vi "Controller.vi"() -> ()   [LabVIEW 2025]
uses:
  Cluster.ctl
  Enum.ctl
  Conn_state.ctl
  <vilib>/Instr/_visa.llb/VISA Configure Serial Port (Instr).vi
  <vilib>/FPGAPlugInAG/myRIO-1900/niLvFpga_Open_myRIO-1900.vi
  <vilib>/rvi/interface/common/dynamic/niFpgaDynamicAddResources.vi
  <vilib>/Utility/error.llb/Error Cluster From Error Code.vi
  <vilib>/rvi/errors/niLvFpgaAdjustHostInterfaceError.vi
  <vilib>/FPGAPlugInAG/Dynamic/niLvFpga_Close_Dynamic.vi
  <vilib>/rvi/interface/nirviOpenFPGA/nirviOpenFPGA.xnode
  FPGA Bitfiles/project_FPGATarget_fpgamain_qld3yE8o4VA.lvbitx
  <vilib>/rvi/interface/nirviReadWriteControl/nirviReadWriteControl.xnode
  <vilib>/rvi/interface/nirviCloseFPGA/nirviCloseFPGA.xnode
  <resource>/objmgr/ni.dex.rc
  <vilib>/rvi/interface/Simulation/niFpgaSimulationCallBeginRW.vi
  NiFpgaLv.dll
panel:
  out "TEMPERATURA":dbl
  in  "Acq_delay_start":u16=500
  out "Is Connected":bool
  out "Stop":bool
  out "Acq_Data":i16[](graph)
  out "error out":errorcluster
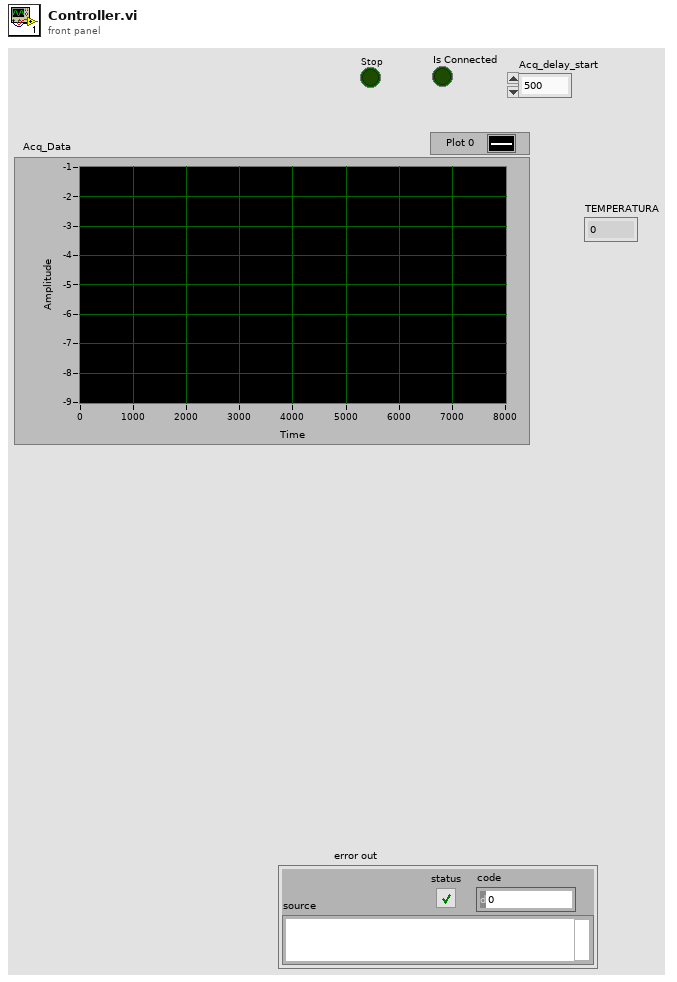
[diagram p1: front panel]
types:
  T1 = typedef "Conn_state.ctl" = enum16{"Disconected", "Reconecting", "Connected"}
  T2 = typedef "Cluster.ctl" = cluster{"Stop":bool, "Trigger":bool, "Select":T3, "Acq Delay":u16}
  T3 = typedef "Enum.ctl" = enum16{"Trigger", "Stop", "Acq_del"}
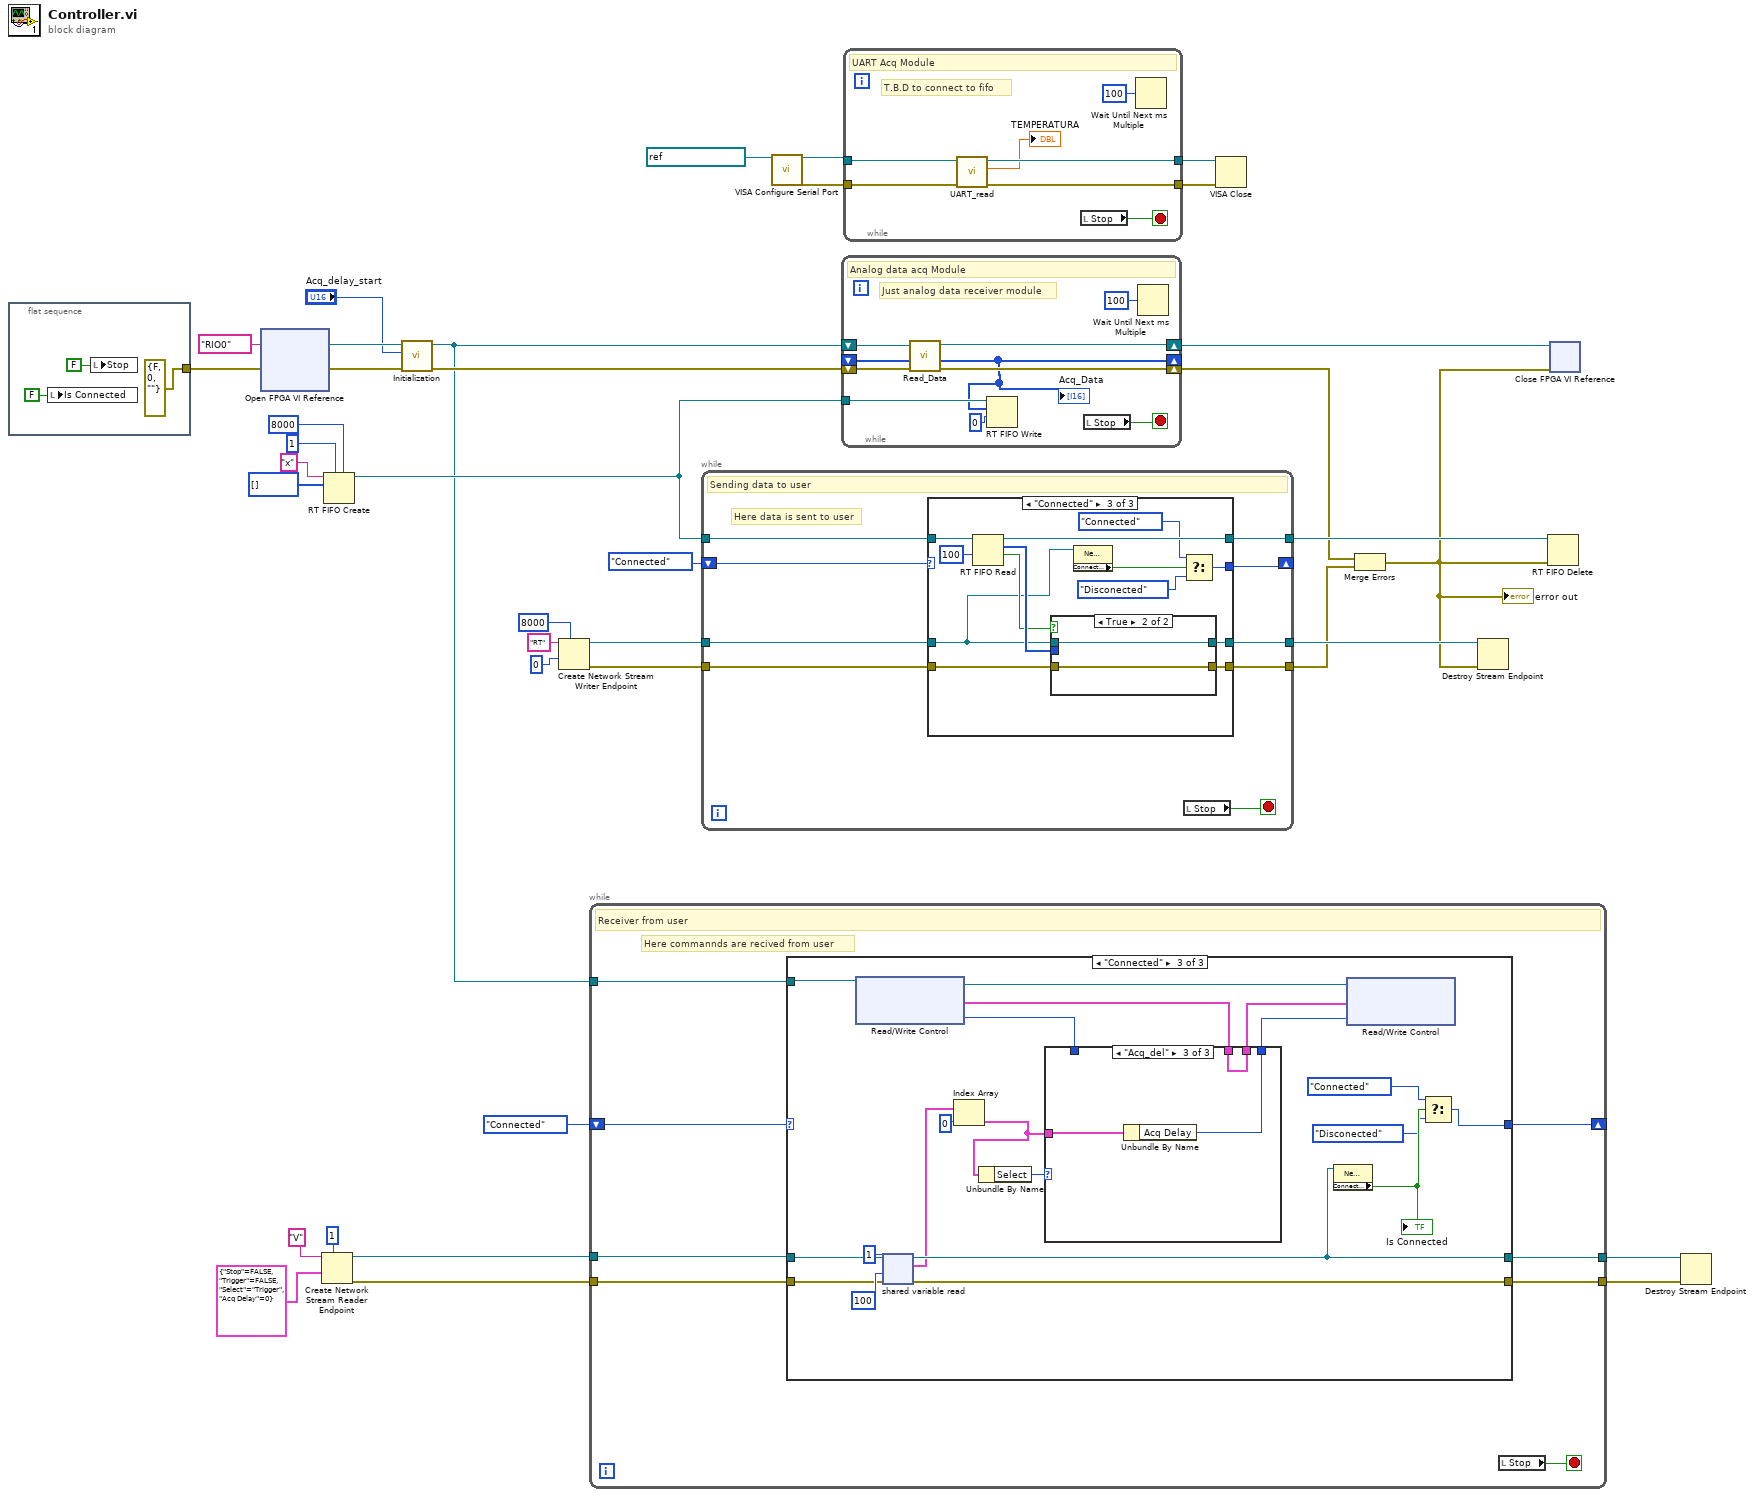
[diagram p0: block diagram]
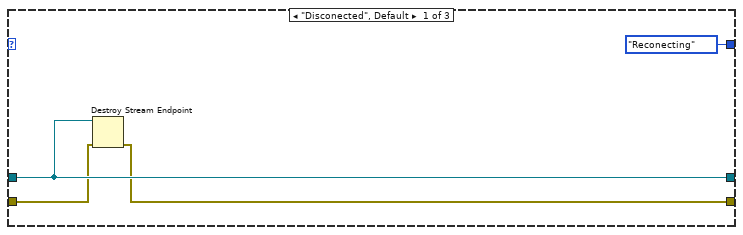
[diagram p2: hidden frame]
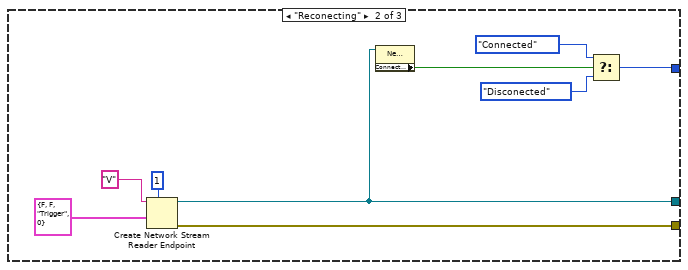
[diagram p3: hidden frame]
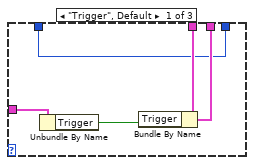
[diagram p4: hidden frame]
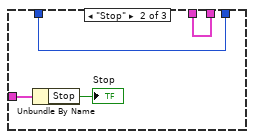
[diagram p5: hidden frame]
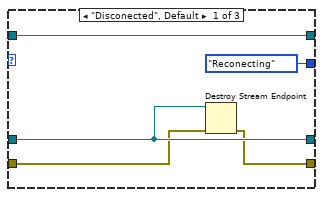
[diagram p6: hidden frame]
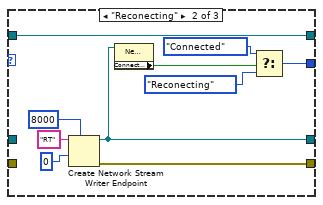
[diagram p7: hidden frame]
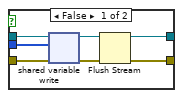
[diagram p8: hidden frame]
diagram:
  n1 = flat-sequence {
    tunnel: [errorcluster {"status"=FALSE, "code"=0, "source"=""} ("error in")] -> w26
    frame #0 {
      n2 = local write "Is Connected"(FALSE ("Is Connected")) -> ()
      n3 = local write "Stop"(FALSE ("Stop")) -> ()
    }
  }
  n4 = xnode "Open FPGA VI Reference"("error in"=w26, "resource name"=tag "RIO0") -> ("FPGA VI Reference Out"=w10:refnum<k20>, "error out"=w29:errorcluster)
  n5 = Create Network Stream Reader Endpoint(7:1 ("reader buffer size"), 9:T2 {"Stop"=FALSE, "Trigger"=FALSE, "Select"=enum."Trigger", "Acq Delay"=0} ("Variable"), 11:"V" ("reader name")) -> (0:w8:errorcluster, 3:w14:refnum<k21>)  [unwired: 4 in]
  n6 = RT FIFO Create(0:"x" ("name (unnamed)"), 1:i32[] [], 4:u32 1 ("size (10)"), 6:u32 8000 ("elements in array (1)")) -> (8:w32:refnum<k33>)  [unwired: 4 in, 2 out]
  n7 = call "Initialization.vi"("error in"=w29, "Acc_delay"="Acq_delay_start", "FPGA VI Reference In"=w10) -> ("error out"=w28:errorcluster, "FPGA VI Reference Out"=w6:refnum<k20>)  [unwired: 7 in]
  n8 = Create Network Stream Writer Endpoint(7:8000 ("writer buffer size"), 9:0, 11:"RT" ("writer name")) -> (0:w19:errorcluster, 3:w21:refnum<k21>)  [unwired: 4 in]
  n9 = while {
    tunnel: w6 -> [w48]
    tunnel: [w45] -> w17
    tunnel: w14 -> [w46]
    shift-right: [w43] -> _
    shift-left: Conn_state."Connected" ("Conn_state") -> [w44]
    tunnel: w8 -> [w42]
    tunnel: [w41] -> w7
    stop <- w47 stop-if-true
    # "Here commannds are recived from user"
    # "Receiver from user"
    n10 = case shown="\"Connected\"" w44 {
      tunnel: w48 -> [_ _ w81]
      tunnel: [w51 w54 w72] -> w45
      tunnel: w46 -> [w51 _ w70]
      tunnel: [Conn_state."Reconecting" ("Conn_state") w58 w66] -> w43
      tunnel: w42 -> [w50 _ w65]
      tunnel: [w49 w53 w64] -> w41
      frame "Disconected", Default {
        n11 = Destroy Stream Endpoint(8:w50, 11:w51) -> (0:w49:errorcluster)
      }
      frame "Reconecting" {
        n12 = Create Network Stream Reader Endpoint(7:1 ("reader buffer size"), 9:T2 {"Stop"=FALSE, "Trigger"=FALSE, "Select"=enum."Trigger", "Acq Delay"=0} ("Variable"), 11:"V" ("reader name")) -> (0:w53:errorcluster, 3:w54:refnum<k21>)  [unwired: 4 in]
        n13 = property class="Network Stream Endpoint"(reference=w54) -> ("Connected"=w59:bool)  [unwired: 1 in, 2 out]
        n14 = Select(t=Conn_state."Connected" ("Conn_state"), s=w59, f=Conn_state."Disconected" ("Conn_state")) -> (s? t:f=w58:T1)
      }
      frame "Connected" {
        n15 = xnode "Read/Write Control"("FPGA VI Reference In"=w81) -> ("FPGA VI Reference Out"=w78:refnum<k20>, "Var data"=w77:cluster{"Placeholder":i16, "Trigger":bool}, "Time Delay_Read"=w63:u16)  [unwired: 1 in, 1 out]
        n16 = shared-variable-read(w70, w65, 100 ("timeout ms (-1)"), 1 ("# elements")) -> (w72:refnum<k21>, w64:errorcluster, w71:T2[])  [unwired: 1 out]
        n17 = Index Array(array=w71, index=0) -> (element=w75:T2)
        n18 = Unbundle By Name(w75) -> ("Select"=w74:T3)
        n19 = case shown="\"Acq_del\"" w74 {
          tunnel: [w84 w88 w92] -> w73
          tunnel: w75 -> [w86 w90 w93]
          tunnel: w77 -> [w83 w88 w92]
          tunnel: w63 -> [w82 w87 _]
          tunnel: [w82 w87 w91] -> w62
          frame "Trigger", Default {
            n20 = Unbundle By Name(w86) -> ("Trigger"=w85:bool)
            n21 = Bundle By Name(cluster=w83, "Trigger"=w85) -> (w84:cluster{"Placeholder":i16, "Trigger":bool})
          }
          frame "Stop" {
            n22 = Unbundle By Name(w90) -> ("Stop"=→"Stop":bool)
          }
          frame "Acq_del" {
            n23 = Unbundle By Name(w93) -> ("Acq Delay"=w91:u16)
          }
        }
        n24 = property class="Network Stream Endpoint"(reference=w72) -> ("Connected"=w69:bool)  [unwired: 1 in, 2 out]
        "Is Connected" <- w69
        n25 = xnode "Read/Write Control"("FPGA VI Reference In"=w78, "Var data"=w73, "Time Delay_Read"=w62) -> ()  [unwired: 1 in, 2 out]
        n26 = Select(t=Conn_state."Connected" ("Conn_state"), s=w69, f=Conn_state."Disconected" ("Conn_state")) -> (s? t:f=w66:T1)
      }
    }
    n27 = local read "Stop"() -> (w47:bool)
  }
  n28 = while {
    tunnel: w32 -> [w102]
    tunnel: [w101] -> w33
    shift-right: [w98] -> _
    shift-left: Conn_state."Connected" ("Conn_state") -> [w99]
    tunnel: w21 -> [w97]
    tunnel: [w96] -> w20
    tunnel: w19 -> [w95]
    tunnel: [w94] -> w18
    stop <- w100 stop-if-true
    # "Here data is sent to user"
    # "Sending data to user"
    n29 = case shown="\"Connected\"" w99 {
      tunnel: w102 -> [w107 w116 w130]
      tunnel: w95 -> [w104 _ w129]
      tunnel: [w105 w108 w128] -> w96
      tunnel: [w107 w116 w127] -> w101
      tunnel: [w103 w109 w126] -> w94
      tunnel: w97 -> [w105 _ w122]
      tunnel: [Conn_state."Reconecting" ("Conn_state") w117 w118] -> w98
      frame "Disconected", Default {
        n30 = Destroy Stream Endpoint(8:w104, 11:w105) -> (0:w103:errorcluster)
      }
      frame "Reconecting" {
        n31 = Create Network Stream Writer Endpoint(7:8000 ("writer buffer size"), 9:0, 11:"RT" ("writer name")) -> (0:w109:errorcluster, 3:w108:refnum<k21>)  [unwired: 4 in]
        n32 = property class="Network Stream Endpoint"(reference=w108) -> ("Connected"=w115:bool)  [unwired: 1 in, 2 out]
        n33 = Select(t=Conn_state."Connected" ("Conn_state"), s=w115, f=Conn_state."Reconecting" ("Conn_state")) -> (s? t:f=w117:T1)
      }
      frame "Connected" {
        n34 = RT FIFO Read(0:w130, 2:100 ("timeout in ms (0)")) -> (8:w127:refnum<k33>, 9:w125:i32[], 10:w123:bool)  [unwired: 2 in, 2 out]
        n35 = case shown="True" w123 {
          tunnel: w125 -> [w137 _]
          tunnel: w129 -> [w134 w138]
          tunnel: w122 -> [w133 w139]
          tunnel: [w132 w139] -> w128
          tunnel: [w131 w138] -> w126
          frame False {
            n36 = shared-variable-write(w133, w134, w137) -> (w136:refnum<k21>, w135:errorcluster)  [unwired: 1 in, 1 out]
            n37 = Flush Stream(8:w135, 11:w136) -> (0:w131:errorcluster, 3:w132:refnum<k21>)  [unwired: 2 in, 1 out]
          }
          frame True {
          }
        }
        n38 = property class="Network Stream Endpoint"(reference=w122) -> ("Connected"=w121:bool)  [unwired: 1 in, 2 out]
        n39 = Select(t=Conn_state."Connected" ("Conn_state"), s=w121, f=Conn_state."Disconected" ("Conn_state")) -> (s? t:f=w118:T1)
      }
    }
    n40 = local read "Stop"() -> (w100:bool)
  }
  n41 = call-poly "VISA Configure Serial Port"("VISA resource name"=refnum<visa-resource-name> "ASRL1::INSTR") -> ("VISA resource name out"=w2:refnum<visa-resource-name>, "error out"=w1:errorcluster)  [unwired: 13 in]
  n42 = while {
    shift-right: [w140] -> w31
    shift-left: w6 -> [w141]
    shift-right: [w147] -> w30
    shift-left: w28 -> [w146]
    tunnel: w32 -> [w148]
    shift-right: [w143] -> _
    shift-left: _ -> [w145]
    stop <- w142 stop-if-true
    # "Just analog data receiver module"
    # "Analog data acq Module"
    n43 = call "Read_Data.vi"("error in"=w146, "Shift_Register_In"=w145, "FPGA VI Reference In"=w141) -> ("error out"=w147:errorcluster, "Shift_Register_Out"=w143:i16[], "FPGA VI Reference Out 2"=w140:refnum<k20>)  [unwired: 6 in]
    "Acq_Data" <- w143
    n44 = RT FIFO Write(0:w148, 1:w143, 2:0 ("timeout in ms (0)")) -> ()  [unwired: 2 in, 4 out]
    n45 = local read "Stop"() -> (w142:bool)
    n46 = Wait Until Next ms Multiple(millisecond multiple=u32 100) -> ()  [unwired: 1 out]
  }
  n47 = while {
    tunnel: w2 -> [w156]
    tunnel: [w155] -> w5
    tunnel: [w154] -> w4
    tunnel: w1 -> [w150]
    stop <- w152 stop-if-true
    # "T.B.D to connect to fifo"
    # "UART Acq Module"
    n48 = call "UART_read.vi"("error in"=w150, "VISA resource name in"=w156) -> ("error out"=w154:errorcluster, "UART_numeric_out"=→"TEMPERATURA":dbl, "VISA resource name out"=w155:refnum<visa-resource-name>)  [unwired: 7 in]
    n49 = local read "Stop"() -> (w152:bool)
    n50 = Wait Until Next ms Multiple(millisecond multiple=u32 100) -> ()  [unwired: 1 out]
  }
  n51 = VISA Close(VISA resource name=w5, error in (no error)=w4) -> ()  [unwired: 1 out]
  n52 = Merge Errors(w30, w18) -> (w11:errorcluster)
  "error out" <- w11
  n53 = Destroy Stream Endpoint(8:w11, 11:w20) -> ()  [unwired: 1 out]
  n54 = RT FIFO Delete(0:w33, 3:w11) -> ()  [unwired: 1 in, 1 out]
  n55 = xnode "Close FPGA VI Reference"("FPGA VI Reference In"=w31, "error in"=w11) -> ()  [unwired: 1 out]
  n56 = Destroy Stream Endpoint(8:w7, 11:w17) -> ()  [unwired: 1 out]
